vi "纳清浊度_所有参数读取.vi"(8 "error in (no error)":errorcluster caption="错误输入（无错误）", 11 "MB session in":refnum<class "MB_Master.lvclass">) -> (0 "error out":errorcluster caption="错误输出", 2 "输出值":T1 {"波特率" items=["4800", "9600", "19200", "38400", "57600", "115200"]}, 3 "MB session out":refnum<class "MB_Master.lvclass">)   [LabVIEW 2016, in "斯坦道多参数.lvlib"]
uses:
  <vilib>/Plasmionique/MB Master/MB_Master/MB_Master.lvclass
  <vilib>/Plasmionique/MB Master/MB Master.lvlib
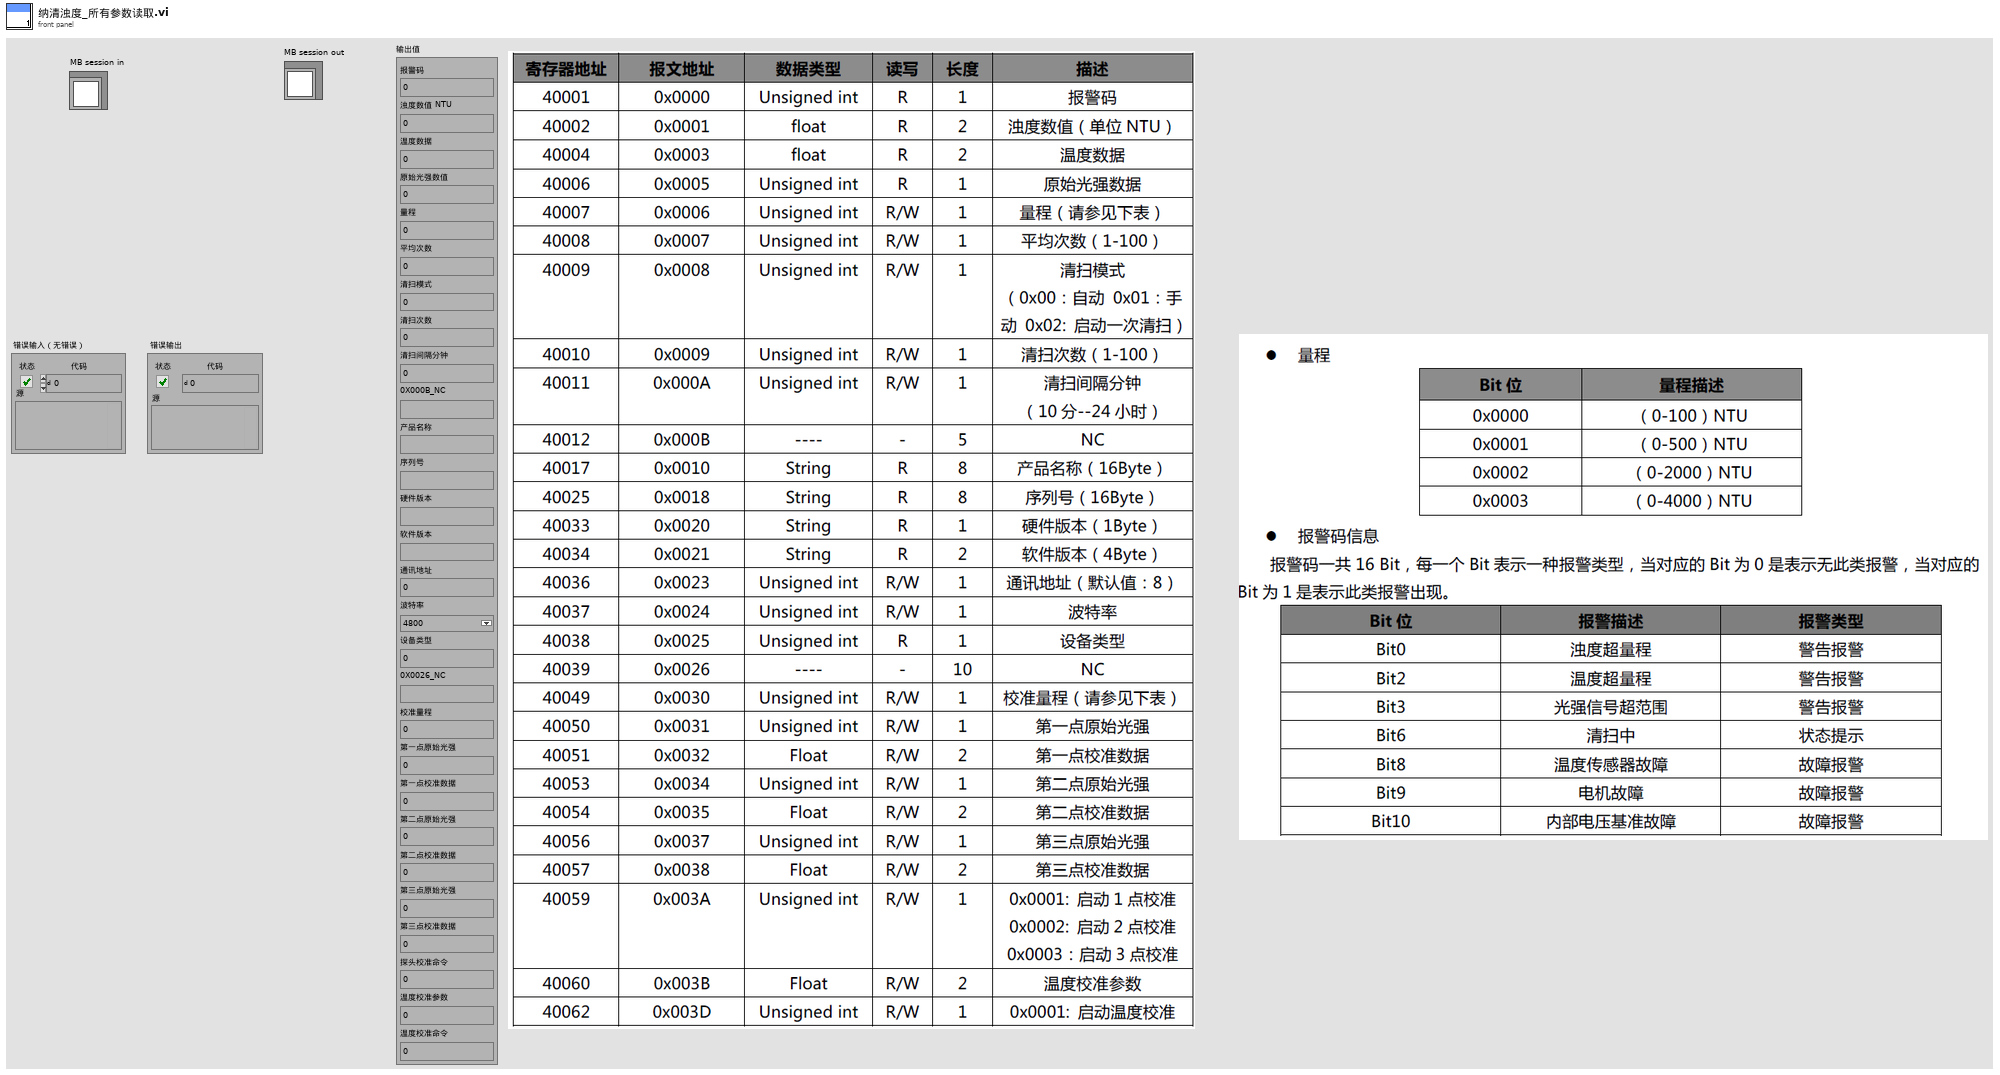
[diagram p1: front panel]
types:
  T1 = cluster{"报警码":u16, "浊度数值 NTU":sgl, "温度数据":sgl, "原始光强数值":u16, "量程":u16, "平均次数":u16, "清扫模式":u16, "清扫次数":u16, "清扫间隔分钟":u16, "0X000B_NC":string, "产品名称":string, "序列号":string, "硬件版本":string, "软件版本":string, "通讯地址":u16, "波特率":u16, "设备类型":u16, "0X0026_NC":string, "校准量程":u16, "第一点原始光强":u16, "第一点校准数据":sgl, "第二点原始光强":u16, "第二点校准数据":sgl, "第三点原始光强":u16, "第三点校准数据":sgl, "探头校准命令":u16, "温度校准参数":sgl, "温度校准命令":u16}
  T2 = cluster{u16, "mode":dbl, "数值":sgl, u16, u16, u16, u16, u16, u16, "类型":string, "类型":string, "类型":string, "类型":string, "类型":string, u16, u16, u16, "类型":string, u16, u16, "数值":sgl, u16, "数值":sgl, u16, "数值":sgl, u16, "数值":sgl, u16}
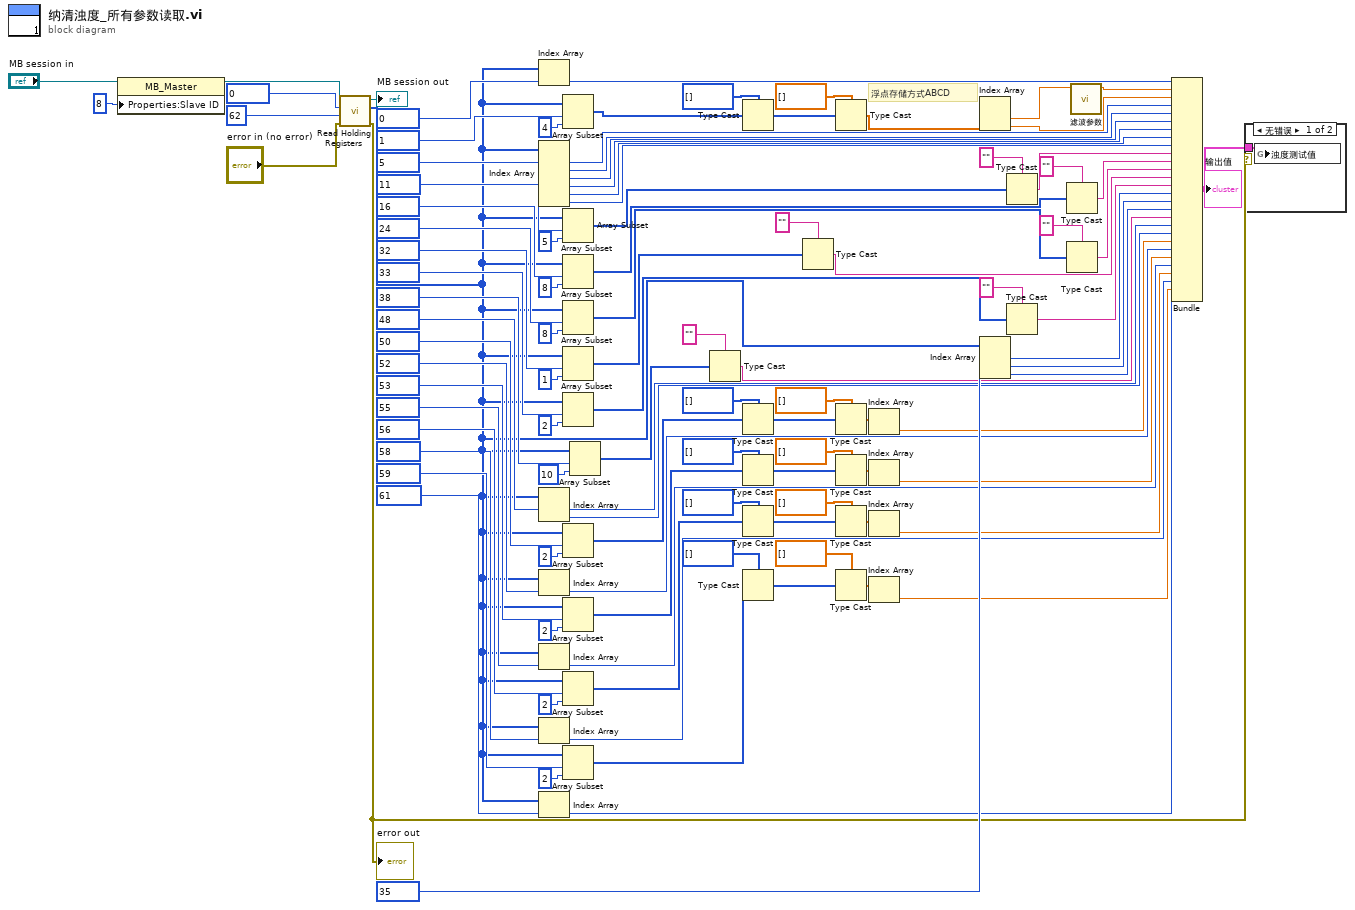
[diagram p0: block diagram]
diagram:
  # "浮点存储方式ABCD"
  n1 = property class="MB_Master"(reference="MB session in", "Properties:Slave ID"=u8 8 ("Slave ID")) -> (reference out=w96:refnum<class "MB_Master.lvclass">)  [unwired: 1 in, 1 out]
  n2 = call <vilib>:"Read Holding Registers.vi"("error in (no error)"="error in (no error)", "quantity"=u16 62, "starting address"=u16 0, "MB session in"=w96) -> ("error out"=w7:errorcluster, "Registers"=w9:u16[], "MB session out"=→"MB session out":refnum<class "MB_Master.lvclass">)  [unwired: 5 in]
  "error out" <- w7
  n3 = Index Array(array=w9, index=u16 0 ("starting address")) -> (element=w104:u16)
  n4 = Index Array(array=w9, index #1=u16 5 ("starting address")) -> (element #1=w91:u16, element #2=w90:u16, element #3=w89:u16, element #4=w88:u16, element #5=w87:u16, element #6=w86:u16)  [unwired: 5 in]
  n5 = Index Array(array=w9, index #1=u16 48 ("starting address")) -> (element #1=w50:u16, element #2=w49:u16)  [unwired: 1 in]
  n6 = Index Array(array=w9, index=u16 52 ("starting address")) -> (element=w32:u16)
  n7 = Index Array(array=w9, index=u16 55 ("starting address")) -> (element=w22:u16)
  n8 = Index Array(array=w9, index=u16 58 ("starting address")) -> (element=w12:u16)
  n9 = Index Array(array=w9, index=u16 61 ("starting address")) -> (element=w8:u16)
  n10 = Array Subset(array=w9, index=u16 1 ("starting address"), length=4 ("长度")) -> (w100:u16[])
  n11 = Array Subset(array=w9, index=u16 11 ("starting address"), length=5 ("长度")) -> (w83:u16[])
  n12 = Array Subset(array=w9, index=u16 16 ("starting address"), length=8 ("长度")) -> (w79:u16[])
  n13 = Array Subset(array=w9, index=u16 24 ("starting address"), length=8 ("长度")) -> (w73:u16[])
  n14 = Array Subset(array=w9, index=u16 32 ("starting address"), length=1 ("长度")) -> (w69:u16[])
  n15 = Array Subset(array=w9, index=u16 33 ("starting address"), length=2 ("长度")) -> (w63:u16[])
  n16 = Array Subset(array=w9, index=u16 50 ("starting address"), length=2 ("长度")) -> (w47:u16[])
  n17 = Array Subset(array=w9, index=u16 53 ("starting address"), length=2 ("长度")) -> (w35:u16[])
  n18 = Array Subset(array=w9, index=u16 56 ("starting address"), length=2 ("长度")) -> (w28:u16[])
  n19 = Array Subset(array=w9, index=u16 59 ("starting address"), length=2 ("长度")) -> (w15:u16[])
  n20 = Array Subset(array=w9, index=u16 38 ("starting address"), length=10 ("长度")) -> (w53:u16[])
  n21 = Type Cast(type="" ("类型"), x=w53) -> (*(type *) &x=w52:string)
  n22 = Type Cast(type=u32[] [] ("数组 2"), x=w100) -> (*(type *) &x=w5:u32[])
  n23 = Type Cast(type=u32[] [] ("数组 2"), x=w47) -> (*(type *) &x=w45:u32[])
  n24 = Type Cast(type=u32[] [] ("数组 2"), x=w35) -> (*(type *) &x=w37:u32[])
  n25 = Type Cast(type=u32[] [] ("数组 2"), x=w28) -> (*(type *) &x=w26:u32[])
  n26 = Type Cast(type=u32[] [] ("数组 2"), x=w15) -> (*(type *) &x=w17:u32[])
  n27 = Type Cast(type="" ("类型"), x=w69) -> (*(type *) &x=w66:string)
  n28 = Type Cast(type=sgl[] [] ("数组 2"), x=w5) -> (*(type *) &x=w99:sgl[])
  n29 = Type Cast(type=sgl[] [] ("数组 2"), x=w45) -> (*(type *) &x=w42:sgl[])
  n30 = Type Cast(type=sgl[] [] ("数组 2"), x=w37) -> (*(type *) &x=w40:sgl[])
  n31 = Type Cast(type=sgl[] [] ("数组 2"), x=w26) -> (*(type *) &x=w23:sgl[])
  n32 = Type Cast(type=sgl[] [] ("数组 2"), x=w17) -> (*(type *) &x=w20:sgl[])
  n33 = Index Array(array=w42) -> (element=w41:sgl)  [unwired: 1 in]
  n34 = Index Array(array=w40) -> (element=w31:sgl)  [unwired: 1 in]
  n35 = Index Array(array=w23) -> (element=w21:sgl)  [unwired: 1 in]
  n36 = Index Array(array=w20) -> (element=w11:sgl)  [unwired: 1 in]
  n37 = Index Array(array=w99) -> (element #1=w2:sgl, element #2=w94:sgl)  [unwired: 2 in]
  n38 = Index Array(array=w9, index #1=u16 35 ("starting address")) -> (element #1=w59:u16, element #2=w58:u16, element #3=w57:u16)  [unwired: 2 in]
  n39 = Type Cast(type="" ("类型"), x=w83) -> (*(type *) &x=w81:string)
  n40 = Type Cast(type="" ("类型"), x=w63) -> (*(type *) &x=w61:string)
  n41 = Type Cast(type="" ("类型"), x=w79) -> (*(type *) &x=w76:string)
  n42 = Type Cast(type="" ("类型"), x=w73) -> (*(type *) &x=w71:string)
  n43 = call "滤波参数.vi"("x"=w2) -> ("mode"=w1:dbl)  [unwired: 10 in]
  n44 = Bundle(w104, "mode"=w1, "数值"=w94, w91, w90, w89, w88, w87, w86, "类型"=w81, "类型"=w76, "类型"=w71, "类型"=w66, "类型"=w61, w59, w58, w57, "类型"=w52, w50, w49, "数值"=w41, w32, "数值"=w31, w22, "数值"=w21, w12, "数值"=w11, w8) -> (w6:T2)  [unwired: 1 in]
  "输出值" <- w6
  n45 = case shown="无错误" w7 {
    tunnel: w6 -> [w107 _]
    frame No Error {
      n46 = global write "纳清过程全局变量.vi" "浊度测试值"(w107) -> ()
    }
    frame Error {
    }
  }
